vi "bld_qry.vi"(6 "N":i32) -> (1 "Parameters":T1[](array[typedef])=[{"parameter name"="SigId", "type"=enum."Long (I32)", "direction"=enum."Input", "value"=variant}, {"parameter name"="DateAndTime", "type"=enum."Date/Time", "direction"=enum."Input", "value"=variant}, {"parameter name"="X0", "type"=enum."Single (SGL)", "direction"=enum."Input", "value"=variant}, {"parameter name"="dX", "type"=enum."Single (SGL)", "direction"=enum."Input", "value"=variant}, {"parameter name"="Y", "type"=enum."Single (SGL)", "direction"=enum."Input", "value"=variant}], 2 "Query":string="insert into Curves values (?,?,?,")   [LabVIEW 2010]
uses:
  <vilib>/Addons/database/Auxilliary.llb/DB Tools Parameter Info.ctl
  <vilib>/addons/database/Auxilliary.llb/DB Tools DataTypes.ctl
  <vilib>/addons/database/Auxilliary.llb/DB Tools Parameter Dir.ctl
  <vilib>/addons/database/NI_Database_API.lvlib
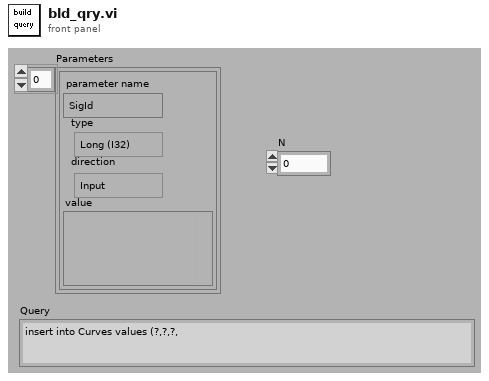
[diagram p1: front panel]
types:
  T1 = typedef "NI_Database_API.lvlib/DB Tools Parameter Info.ctl" = cluster{"parameter name":string, "type":T2, "direction":T3, "value":variant}
  T2 = typedef "NI_Database_API.lvlib/DB Tools DataTypes.ctl" = enum16{"String", "Long (I32)", "Single (SGL)", "Double (DBL)", "Date/Time", "Binary"}
  T3 = typedef "NI_Database_API.lvlib/DB Tools Parameter Dir.ctl" = enum32{"Input", "Output", "Input/Output", "Return Value"}
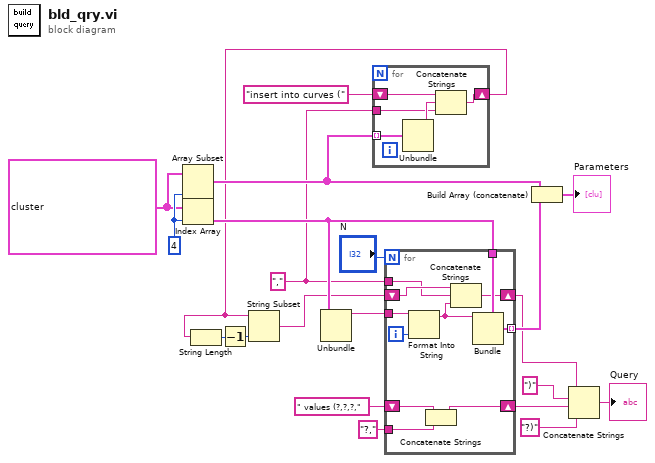
[diagram p0: block diagram]
diagram:
  w6 = ","
  w21 = 4 ("index")
  w20 = T1[] [{"parameter name"="sigid", "type"=enum."Long (I32)", "direction"=enum."Input", "value"=variant}, {"parameter name"="DateAndTime", "type"=enum."Date/Time", "direction"=enum."Input", "value"=variant}, {"parameter name"="X0", "type"=enum."Single (SGL)", "direction"=enum."Input", "value"=variant}, {"parameter name"="dX", "type"=enum."Single (SGL)", "direction"=enum."Input", "value"=variant}, {"parameter name"="Y", "type"=enum."Single (SGL)", "direction"=enum."Input", "value"=variant}] ("parameters")
  n1 = Array Subset(array=w20, length=w21) -> (w8:T1[])  [unwired: 1 in]
  n2 = Index Array(array=w20, index=w21) -> (element=w15:T1)
  n3 = Unbundle(w15) -> ("parameter name"=w19:string)  [unwired: 3 out]
  n4 = for {
    tunnel: w8 -> [w26] mode=indexing
    shift-right: [w24] -> w3
    shift-left: "insert into curves (" -> [w23]
    tunnel: w6 -> [w22]
    n5 = Unbundle(w26) -> ("parameter name"=w25:string)  [unwired: 3 out]
    n6 = Concatenate Strings(w23, w25, w22) -> (w24:string)
  }
  n7 = String Length(string=w3) -> (length=w5:i32)
  n8 = Decrement(x=w5) -> (x-1=w4:i32)
  n9 = String Subset(string=w3, length (rest)=w4) -> (substring=w2:string)  [unwired: 1 in]
  n10 = for {
    N: "N" -> [_]
    tunnel: w15 -> [w37]
    tunnel: [w36] -> w14 mode=indexing
    tunnel: w19 -> [w34]
    shift-right: [w33] -> w17
    shift-left: " values (?,?,?," -> [w32]
    tunnel: "?," -> [w31]
    shift-right: [w29] -> w11
    shift-left: w2 -> [w28]
    tunnel: w6 -> [w27]
    i -> [w35]
    n11 = Format Into String(initial string=w34, w35) -> (resulting string=w30:string)  [unwired: 2 in, 1 out]
    n12 = Concatenate Strings(w32, w31) -> (w33:string)
    n13 = Concatenate Strings(w28, w27, w30) -> (w29:string)
    n14 = Bundle(cluster=w37, "parameter name"=w30) -> (w36:T1)  [unwired: 3 in]
  }
  n15 = Build Array (concatenate)(w8, w14) -> (→"Parameters":T1[])
  n16 = Concatenate Strings(w11, ")" ("string"), w17, "?)" ("string")) -> (→"Query":string)
